vi "testClassCreate.vi"(8 "error in (no error)":errorcluster caption="Fehler (Eingang, kein Fehler)", 11 "test Eingang":refnum<class "test.lvclass"> caption="DNL_LabVIEW Object in") -> (0 "error out":errorcluster caption="Fehler (Ausgang)", 3 "test Ausgang":refnum<class "test.lvclass"> caption="DNL_LabVIEW Object out")   [LabVIEW 2013, in "test.lvclass"]
uses:
  test.lvclass
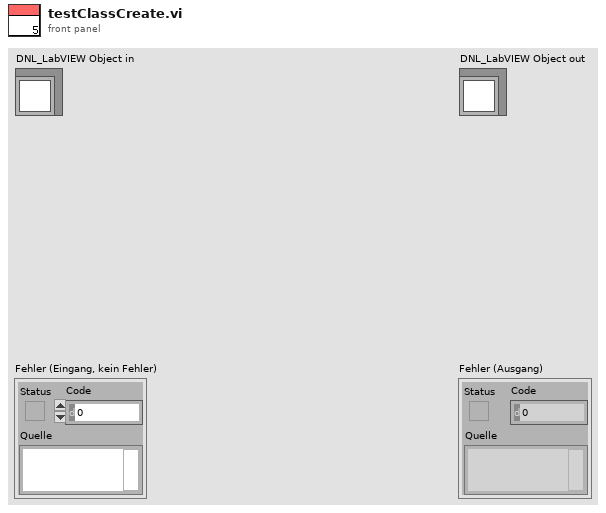
[diagram p1: front panel]
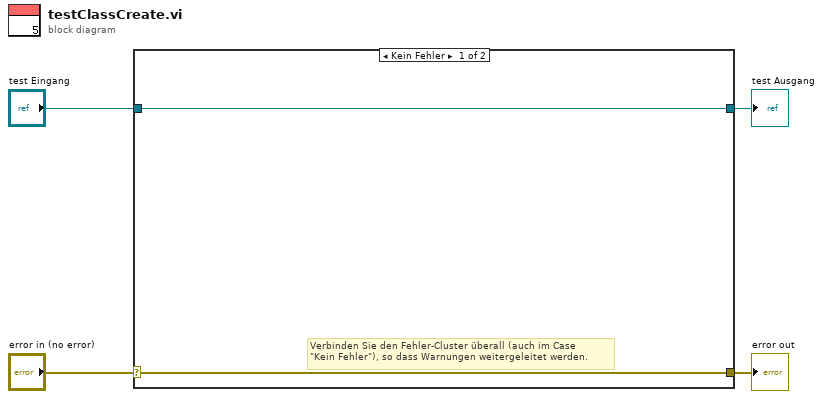
[diagram p0: block diagram]
diagram:
  n1 = case shown="Kein Fehler" "error in (no error)" {
    selector: "error in (no error)" -> [w5 w8]
    tunnel: [w5 w8] -> w3
    tunnel: [w6 w7] -> w1
    tunnel: "test Eingang" -> [w6 w7]
    frame No Error {
      # "Verbinden Sie den Fehler-Cluster überall (auch im Case\n\"Kein Fehler\"), so dass Warnungen weitergeleitet werden."
    }
    frame Error {
    }
  }
  "error out" <- w3
  "test Ausgang" <- w1
